vi "StringTest.vi"(11 "Chaîne":string) -> (3 "Chaîne":string, 5 "abc ?":bool)   [LabVIEW 2020]
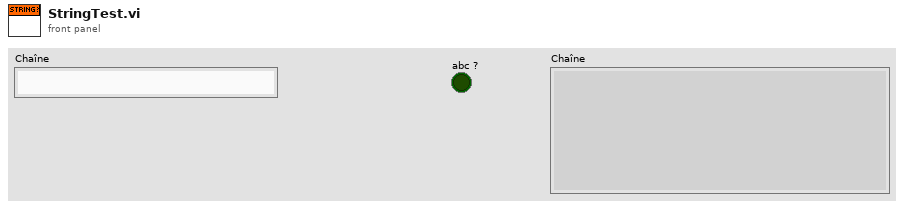
[diagram p1: front panel]
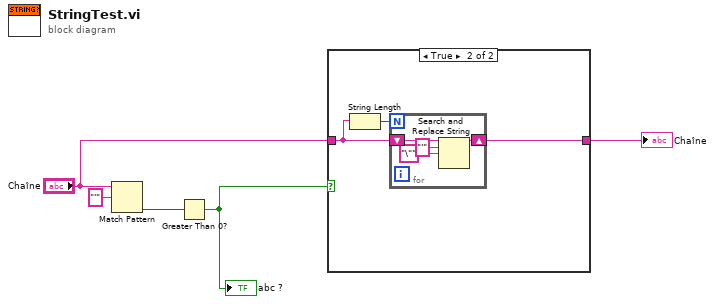
[diagram p0: block diagram]
diagram:
  n1 = Match Pattern(string="Chaîne", regular expression="'" ("expression régulière")) -> (offset past match=w4:i32)  [unwired: 1 in, 3 out]
  n2 = Greater Than 0?(x=w4) -> (x > 0?=w3:bool)
  "abc ?" <- w3
  n3 = case shown="True" w3 {
    tunnel: [w6 w9] -> w2
    tunnel: "Chaîne" -> [w6 w7]
    frame False {
    }
    frame True {
      n4 = String Length(string=w7) -> (length=w8:i32)
      n5 = for {
        N: w8 -> [_]
        shift-right: [w11] -> w9
        shift-left: w7 -> [w10]
        n6 = Search and Replace String(input string=w10, search string="'" ("chaîne recherchée"), replace string="\"" ("chaîne de remplacement (\"\")")) -> (result string=w11:string)  [unwired: 5 in, 3 out]
      }
    }
  }
  "Chaîne" <- w2
